vi "Edge Split Test.vi"() -> ()   [LabVIEW 2016]
panel:
  out "Array":cluster{"Array":dbl[]}[](array[cluster])
  in  "Output values in":dbl[](array[numeric])=[1.0, 2.0, 3.0, 4.0, 5.0, 6.0, 7.0, 8.0, 9.0, 10.0]
  in  "Edge indexies":i32[](array[numeric])
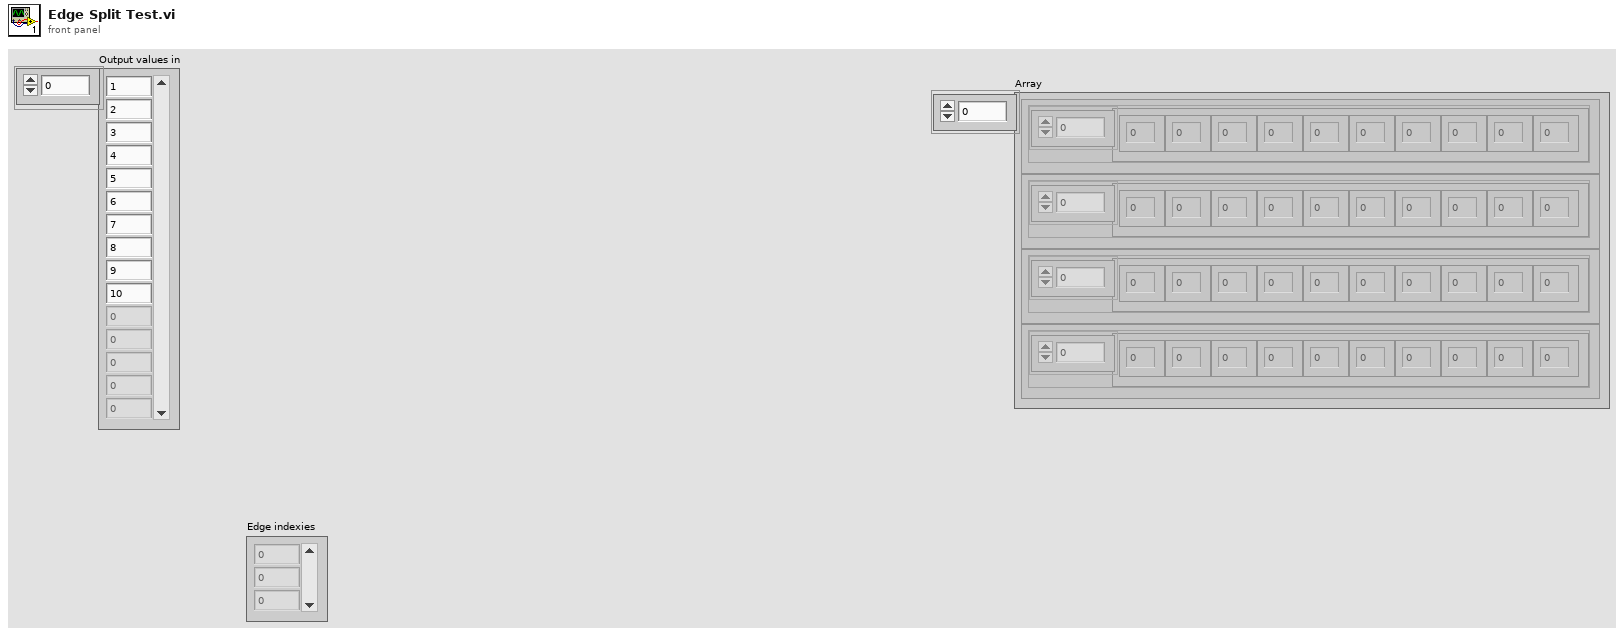
[diagram p1: front panel]
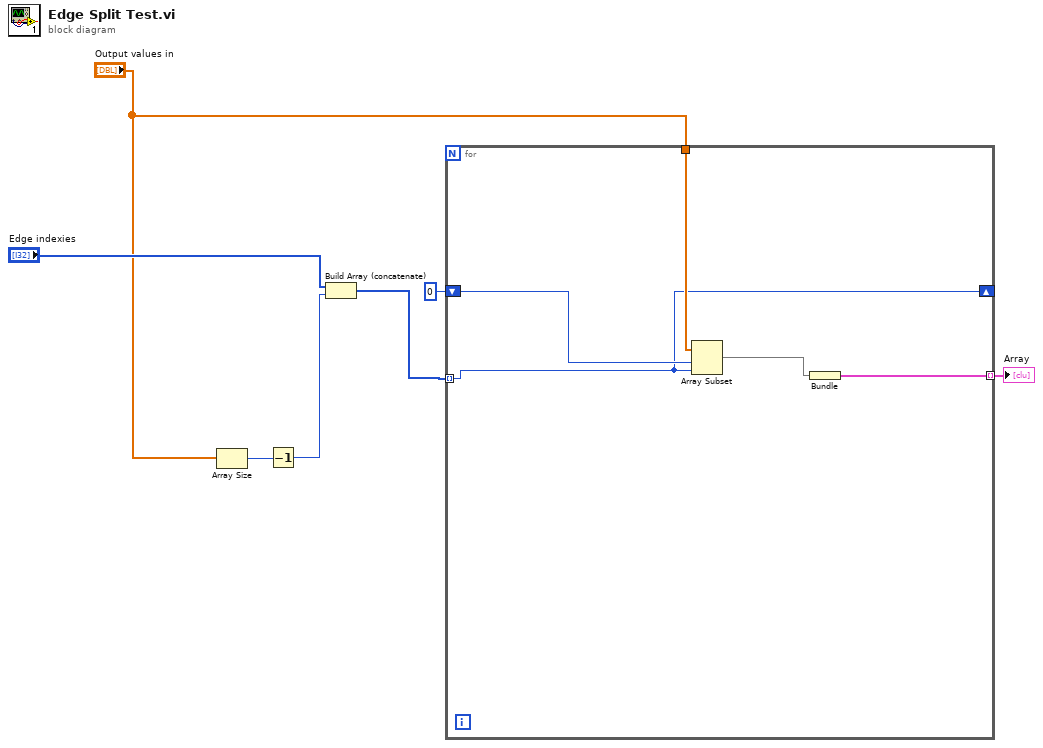
[diagram p0: block diagram]
diagram:
  n1 = Array Size(array="Output values in") -> (size(s)=w6:i32)
  n2 = Decrement(x=w6) -> (x-1=w1:i32)
  n3 = Build Array (concatenate)("Edge indexies", w1) -> (w5:i32[])
  n4 = for {
    shift-right: [w10] -> _
    shift-left: 0 ("Numeric") -> [w11]
    tunnel: w5 -> [w10] mode=indexing
    tunnel: "Output values in" -> [w12]
    tunnel: [w8] -> w2 mode=indexing
    n5 = Array Subset(array=w12, index=w11, length=w10) -> (w9:dbl[])
    n6 = Bundle(w9) -> (w8:cluster{dbl[]})  [unwired: 1 in]
  }
  "Array" <- w2
